vi "CCD Example 2.vi"(8 "error in":errorcluster) -> (0 "error out":errorcluster, 2 "ExposureTime [ms]":i32, 4 "results-JSON string 2":string, 5 "results-JSON string":string)   [LabVIEW 2023]
uses:
  Source/Classes/CCD/CCD.lvclass
  Source/Libraries/DeviceManager/DeviceManager.lvlib
panel:
  out "chip size, y":i32
  out "chip size, x":i32
  # "Connector Pane"
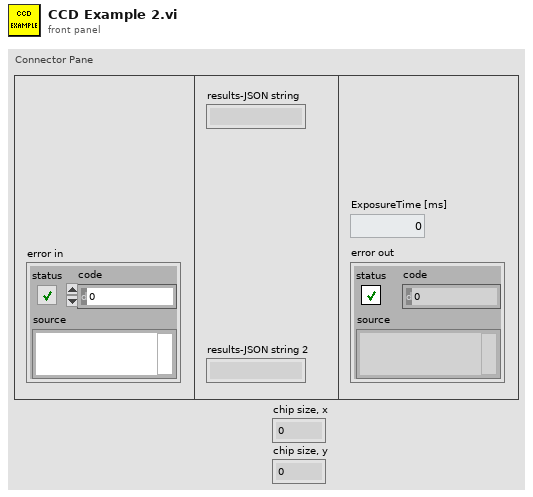
[diagram p1: front panel]
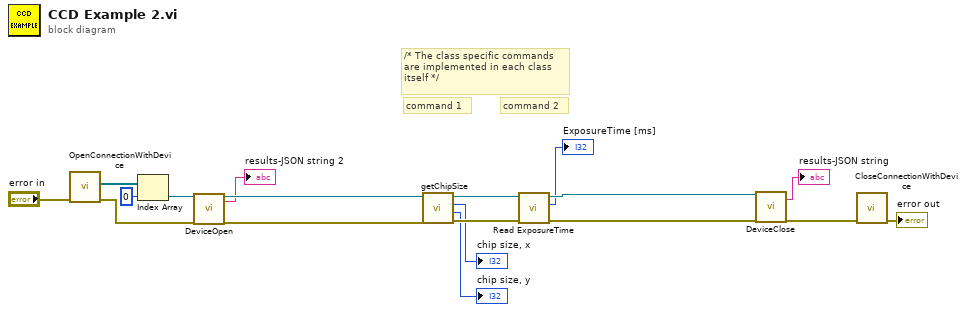
[diagram p0: block diagram]
diagram:
  # "command 2"
  # "command 1"
  # "/* The class specific commands\nare implemented in each class\nitself */"
  n1 = call "OpenConnectionWithDevice.vi"("error in"="error in") -> ("error out"=w10:errorcluster, "CCDs"=w12:refnum<class "CCD.lvclass">[])  [unwired: 7 in, 2 out]
  n2 = Index Array(array=w12, index=0) -> (element=w18:refnum<class "CCD.lvclass">)
  n3 = call-dynamic "DeviceOpen.vi"("CCD in"=w18, "error in (no error)"=w10) -> ("CCD out"=w11:refnum<class "CCD.lvclass">, "results-JSON string"=→"results-JSON string 2":string, "error out"=w17:errorcluster)  [unwired: 12 in, 3 out]
  n4 = call-dynamic "getChipSize.vi"("error in (no error)"=w17, "CCD in"=w11) -> ("error out"=w14:errorcluster, "chip size, y"=→"chip size, y":i32, "chip size, x"=→"chip size, x":i32, "CCD out"=w16:refnum<class "CCD.lvclass">)  [unwired: 6 in]
  n5 = call-dynamic "Read ExposureTime.vi"("error in (no error)"=w14, "CCD in"=w16) -> ("error out"=w13:errorcluster, "ExposureTime [ms]"=→"ExposureTime [ms]":i32, "CCD out"=w15:refnum<class "CCD.lvclass">)  [unwired: 7 in]
  n6 = call-dynamic "DeviceClose.vi"("CCD in"=w15, "error in (no error)"=w13) -> ("results-JSON string"=→"results-JSON string":string, "error out"=w8:errorcluster)  [unwired: 12 in, 4 out]
  n7 = call "CloseConnectionWithDevice.vi"("error in (no error)"=w8) -> ("error out"=→"error out":errorcluster)  [unwired: 10 in]
